vi "Process.vi"(0 "Process In":refnum<class "Process Handler.lvclass">, 11 "Error In":errorcluster) -> (4 "Process Out":refnum<class "Process Handler.lvclass">, 15 "Error Out":errorcluster)   [LabVIEW 2023, in "Process Handler.lvclass"]
uses:
  Process Handler.lvclass
  H:/Desktop/LabVIEW/LabView Repo/LabVIEW-Class-Framework/Classes/Processes/Process/Process.lvclass
  Private/Ctrls/Process Variables.ctl
  Process/Process.lvclass
  H:/Desktop/LabVIEW/LabView Repo/LabVIEW-Class-Framework/Interfaces/ICanCommunicate/ICanCommunicate.lvclass
  Interfaces/ICanCommunicate/Message.ctl
  Message Handler/Message Handler.lvclass
  Process Handler.lvclass/Process Handler.ctl
  Interfaces/ICanCommunicate/ICanCommunicate.lvclass
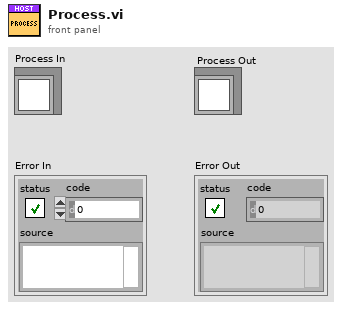
[diagram p1: front panel]
types:
  T1 = typedef "ICanCommunicate.lvclass/Message.ctl" = cluster{"Sender Name":string, "Recipent Name":string, "Command":string, "Data":variant, "Time Stamp":timestamp, "GUID":string, "Chcecksum":string}
  T2 = typedef "Process Handler.lvclass/Process Variables.ctl" = cluster{"Spawn Processes":refnum<class "Process.lvclass">[]}
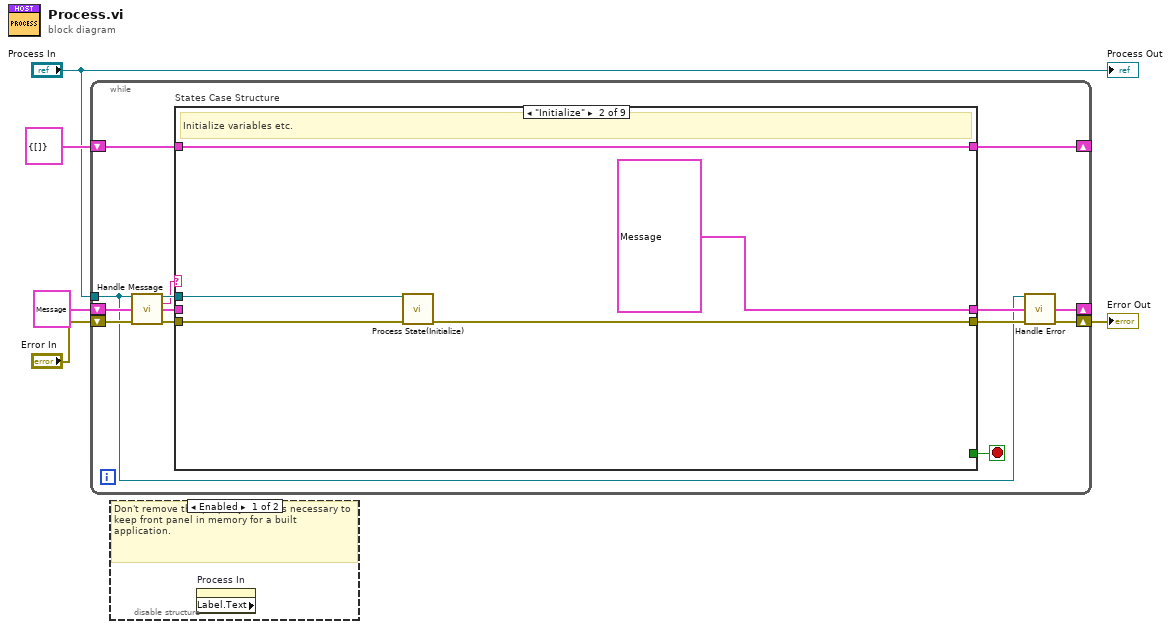
[diagram p0: block diagram]
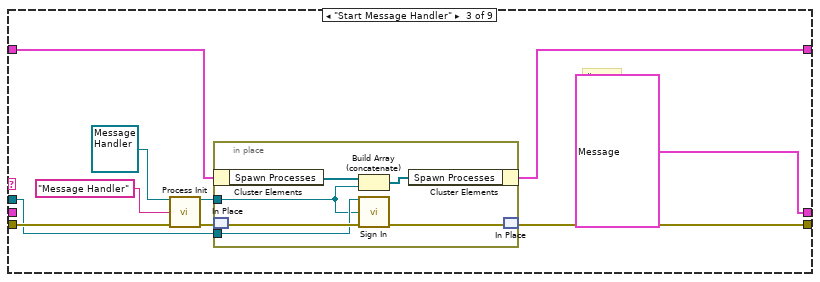
[diagram p3: hidden frame]
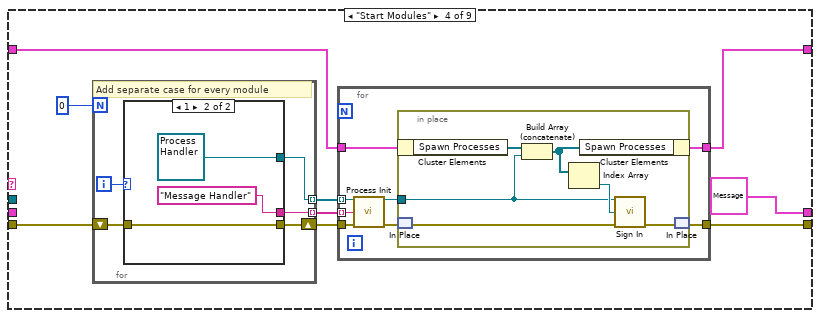
[diagram p4: hidden frame]
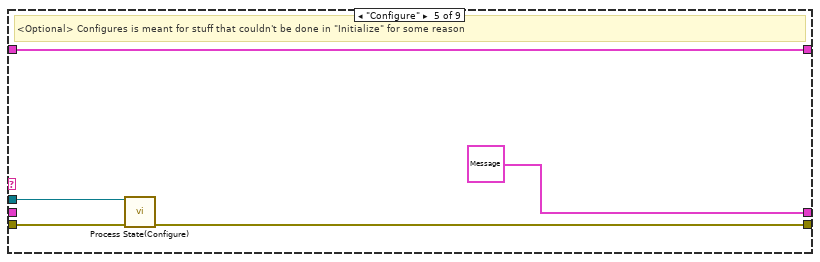
[diagram p6: hidden frame]
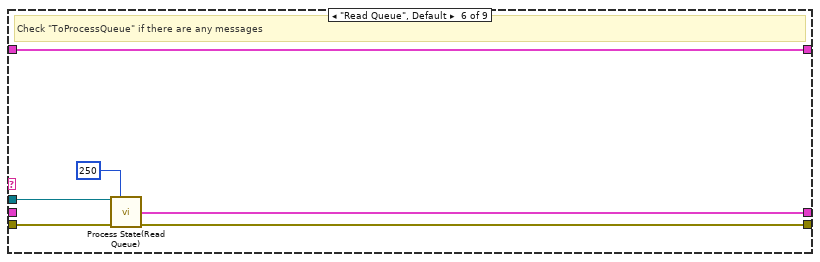
[diagram p7: hidden frame]
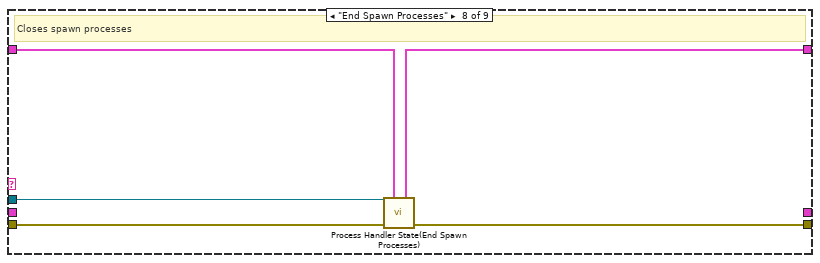
[diagram p9: hidden frame]
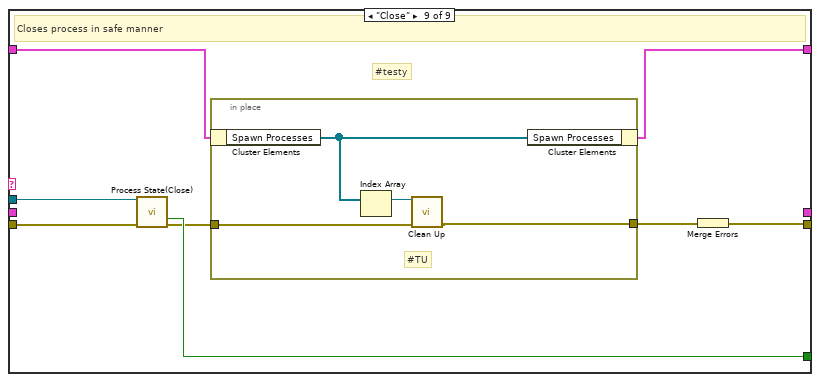
[diagram p10: hidden frame]
diagram:
  n1 = while {
    shift-right: [w9] -> w5
    shift-left: "Error In" -> [w15]
    tunnel: "Process In" -> [w6]
    shift-right: [w18] -> _
    shift-left: T2 {"Spawn Processes"=[]} ("Process Variables") -> [w17]
    shift-right: [w7] -> _
    shift-left: T1 {"Sender Name"="", "Recipent Name"="", "Command"="Initialize", "Data"=variant, "Time Stamp"=timestamp(0 s since 1904-01-01), "GUID"="", "Chcecksum"=""} ("Message") -> [w12]
    stop <- w16 stop-if-true
    n2 = call-dynamic "Handle Message.vi"("ICanComunicate In"=w6, "Message In"=w12, "Error In"=w15) -> ("ICanComunicate Out"=w11:refnum<class "Process Handler.lvclass">, "CMD Out"=w10:string, "Message Out"=w13:T1, "Error Out"=w14:errorcluster)  [unwired: 9 in]
    n3 = case "States Case Structure" shown="\"Initialize\"" w10 {
      tunnel: w14 -> [w22 w26 w37 w46 w77 w84 w88 w89 w101]
      tunnel: [w22 w24 w31 w47 w75 w83 w88 w91 w94] -> w19
      tunnel: [w21 w27 w32 w48 w79 w85 w87 w92 w96] -> w18
      tunnel: w17 -> [w21 w27 w33 w49 w79 w85 w87 w93 w98]
      tunnel: [_ _ _ _ _ _ _ _ w99] -> w16
      tunnel: w13 -> [w20 _ _ _ _ _ w86 _ _]
      tunnel: [w20 T1 {"Sender Name"="", "Recipent Name"="", "Command"="Start Message Handler", "Data"=variant, "Time Stamp"=timestamp(0 s since 1904-01-01), "GUID"="", "Chcecksum"=""} ("Message") T1 {"Sender Name"="", "Recipent Name"="", "Command"="Read Queue", "Data"=variant, "Time Stamp"=timestamp(0 s since 1904-01-01), "GUID"="", "Chcecksum"=""} ("Message") T1 {"Sender Name"="", "Recipent Name"="", "Command"="Read Queue", "Data"=variant, "Time Stamp"=timestamp(0 s since 1904-01-01), "GUID"="", "Chcecksum"=""} ("Message") T1 {"Sender Name"="", "Recipent Name"="", "Command"="Read Queue", "Data"=variant, "Time Stamp"=timestamp(0 s since 1904-01-01), "GUID"="", "Chcecksum"=""} ("Message") w82 w86 _ _] -> w8
      tunnel: w11 -> [_ w25 w28 _ w76 w81 _ w90 w100]
      frame "--- Common ---" {
        # "Only for grouping"
      }
      frame "Initialize" {
        # "Initialize variables etc."
        n4 = call-dynamic "Process State(Initialize).vi"("Process In"=w25, "Error In"=w26) -> ("Error Out"=w24:errorcluster)  [unwired: 12 in, 1 out]
      }
      frame "Start Message Handler" {
        # "#testy"
        n5 = call-dynamic "Process Init.vi"("Process In"=refnum<class "Message Handler.lvclass"> refnum ("Process"), "Process Name"="Message Handler" ("Process ID"), "Error In"=w37) -> ("Process Out"=w30:refnum<class "Message Handler.lvclass">, "Error Out"=w29:errorcluster)  [unwired: 11 in]
        n6 = in-place {
          in-place-border: w30 -> [w38]
          in-place-border: w28 -> [w41]
          n7 = in-place-cluster #1(w33) -> ("Spawn Processes"=w39:refnum<class "Process.lvclass">[])
          n8 = in-place-match #2(w29) -> (w43:errorcluster)
          n9 = Build Array (concatenate)(w39, w38) -> (w40:refnum<class "Process.lvclass">[])
          n10 = call-dynamic "Sign In.vi"("ICanCommunicate In"=w41, "Message Handler"=w38, "Error In"=w43) -> ("Error Out"=w42:errorcluster)  [unwired: 11 in, 1 out]
          n11 = in-place-cluster #1("Spawn Processes"=w40) -> (w32:T2)
          n12 = in-place-match #2(w42) -> (w31:errorcluster)
        }
      }
      frame "Start Modules" {
        n13 = for {
          N: 0 -> [_]
          tunnel: [w71] -> w52 mode=indexing
          tunnel: [w70] -> w51 mode=indexing
          shift-right: [w68] -> w45
          shift-left: w46 -> [w69]
          i -> [w67]
          # "Add separate case for every module"
          n14 = case shown="1" w67 {
            tunnel: [_ refnum<class "Process Handler.lvclass"> refnum ("Process")] -> w71
            tunnel: [_ "Message Handler" ("Process ID")] -> w70
            tunnel: w69 -> [_ w72]
            tunnel: [_ w72] -> w68
            frame 0, Default {
            }
            frame 1 {
            }
          }
        }
        n15 = for {
          tunnel: w52 -> [w60] mode=indexing
          tunnel: w51 -> [w59] mode=indexing
          tunnel: w49 -> [w58]
          tunnel: [w57] -> w48
          tunnel: [w56] -> w47
          tunnel: w45 -> [w53]
          n16 = call-dynamic "Process Init.vi"("Process In"=w60, "Process Name"=w59, "Error In"=w53) -> ("Process Out"=w55:refnum<class "Process Handler.lvclass">, "Error Out"=w54:errorcluster)  [unwired: 11 in]
          n17 = in-place {
            in-place-border: w55 -> [w62]
            n18 = in-place-cluster #3(w58) -> ("Spawn Processes"=w64:refnum<class "Process.lvclass">[])
            n19 = in-place-match #4(w54) -> (w66:errorcluster)
            n20 = Build Array (concatenate)(w64, w62) -> (w61:refnum<class "Process.lvclass">[])
            n21 = Index Array(array=w61) -> (element=w63:refnum<class "Process.lvclass">)  [unwired: 1 in]
            n22 = in-place-cluster #3("Spawn Processes"=w61) -> (w57:T2)
            n23 = call-dynamic "Sign In.vi"("ICanCommunicate In"=w62, "Message Handler"=w63, "Error In"=w66) -> ("Error Out"=w65:errorcluster)  [unwired: 11 in, 1 out]
            n24 = in-place-match #4(w65) -> (w56:errorcluster)
          }
        }
      }
      frame "Configure" {
        # "<Optional> Configures is meant for stuff that couldn't be done in \"Initialize\" for some reason"
        n25 = call-dynamic "Process State(Configure).vi"("Process In"=w76, "Error In"=w77) -> ("Error Out"=w75:errorcluster)  [unwired: 12 in, 1 out]
      }
      frame "Read Queue", Default {
        # "Check \"ToProcessQueue\" if there are any messages"
        n26 = call-dynamic "Process State(Read Queue).vi"("Process In"=w81, "Timeout in ms (-1)"=250, "Error In"=w84) -> ("Message"=w82:T1, "Error Out"=w83:errorcluster)  [unwired: 9 in, 2 out]
      }
      frame "Timeout" {
        # "<Optional> Actions to be taken if there are no messages for process"
      }
      frame "End Spawn Processes" {
        # "Closes spawn processes"
        n27 = call "Process Handler State(End Spawn Processes).vi"("Process Handler In"=w90, "Process Variables In"=w93, "Error In"=w89) -> ("Process Variables Out"=w92:T2, "Error Out"=w91:errorcluster)  [unwired: 10 in, 1 out]
      }
      frame "Close" {
        # "#testy"
        # "Closes process in safe manner"
        n28 = call-dynamic "Process State(Close).vi"("Process In"=w100, "Error In"=w101) -> ("Close?"=w99:bool, "Error Out"=w97:errorcluster)  [unwired: 11 in, 1 out]
        n29 = in-place {
          in-place-border: w97 -> [w105]
          in-place-border: [w104] -> w95
          # "#TU"
          n30 = in-place-cluster #5(w98) -> ("Spawn Processes"=w103:refnum<class "Process.lvclass">[])
          n31 = Index Array(array=w103) -> (element=w102:refnum<class "Process.lvclass">)  [unwired: 1 in]
          n32 = call-dynamic "Clean Up.vi"("Process In"=w102, "Error In"=w105) -> ("Error Out"=w104:errorcluster)  [unwired: 12 in, 1 out]
          n33 = in-place-cluster #5("Spawn Processes"=w103) -> (w96:T2)
        }
        n34 = Merge Errors(w95) -> (w94:errorcluster)
      }
    }
    n35 = call-dynamic "Handle Error.vi"("Process In"=w6, "Message In"=w8, "Error In"=w19) -> ("Message Out"=w7:T1, "Error Out"=w9:errorcluster)  [unwired: 10 in, 1 out]
  }
  "Error Out" <- w5
  n36 = disable-structure shown="Enabled" {
    frame Enabled {
      # "Don't remove this property node it's necessary to keep front panel in memory for a built application."
      n37 = property on="Process In" class="LVClassControl (strict)" props=["Label", "Text"]() -> ()  [unwired: 2 in, 3 out]
    }
    frame Disabled {
    }
  }
  "Process Out" <- "Process In"
